vi "uc480_Sharpness_Measurement.vi"() -> ()   [LabVIEW 2011]
uses:
  C:/Program Files/Thorlabs/Scientific Imaging/DCx Camera Support/Develop/DotNet/uc480DotNet.dll
  Develop/DotNet/uc480DotNet.dll
panel:
  in  "Measuring Region":u32(ring) items=["Center", "Upper Left", "Upper Right", "Lower Left", "Lower Right"]
  in  "Zoom":enum32{"1:4", "1:2", "1:1", "2:1"}(radio)
  out "Sharpness":u32(slide) scale=0.0..100.0
  out "Image":picture
  in  "Camera ID":i32 min=0 max=255
  out "Serial Number":string
  out "AOI Height":i32=8
  out "AOI Width":i32=8
  out "Bits/Pixel":i32=8
  out "Error Out":errorcluster caption="error"
  in  "Exit Camera":bool
  in  "Init Camera":bool
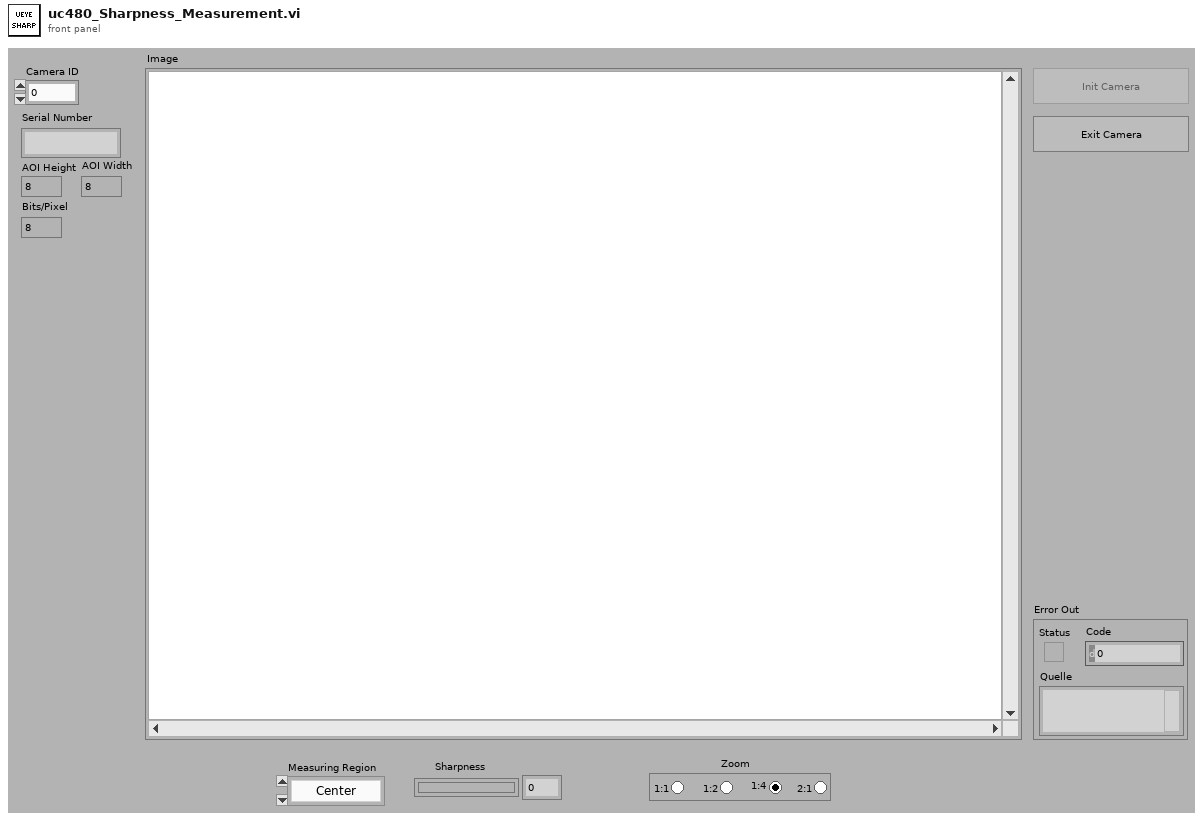
[diagram p1: front panel]
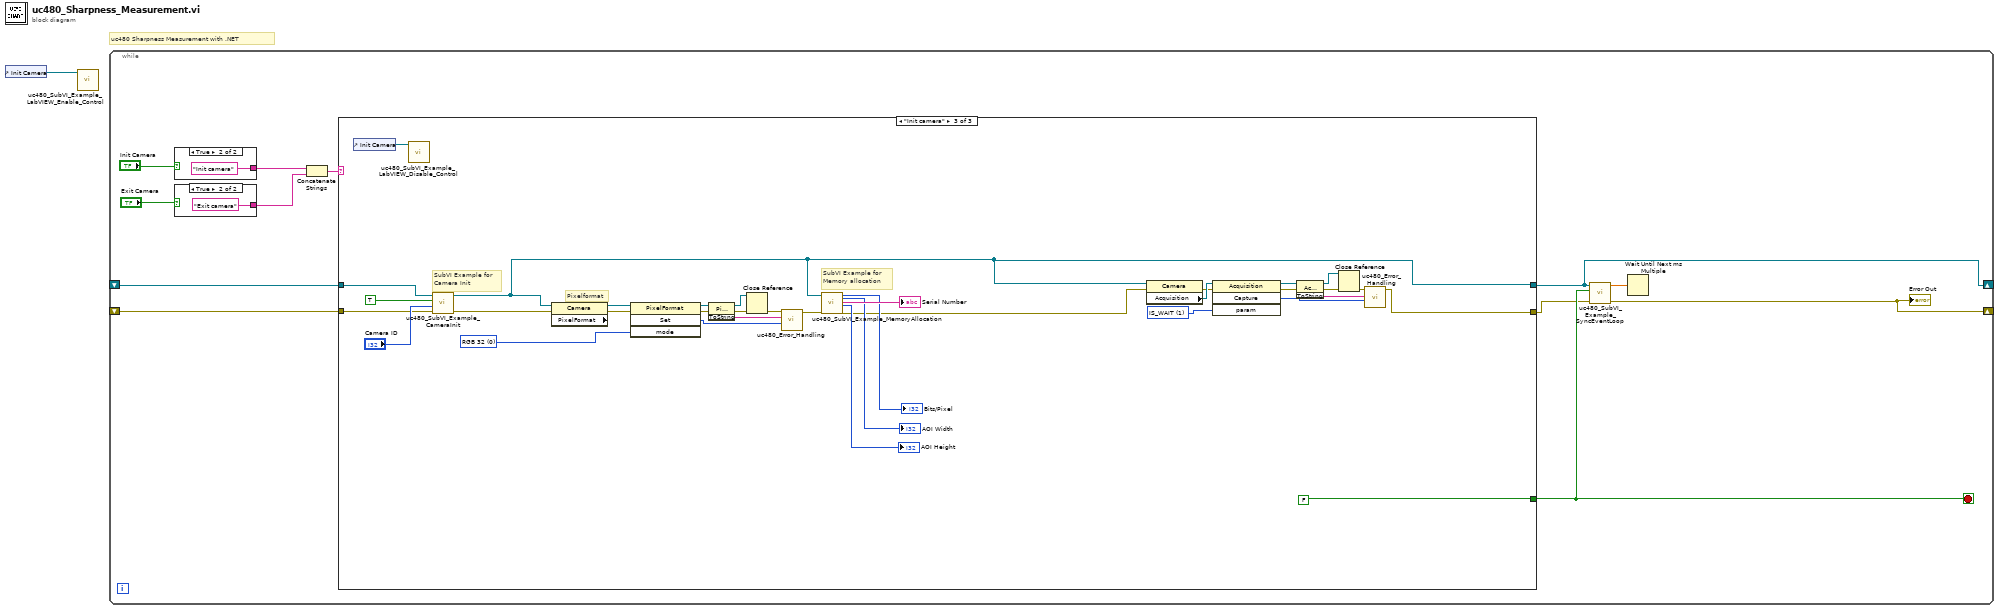
[diagram p0: block diagram]
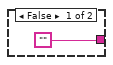
[diagram p2: hidden frame]
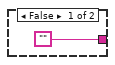
[diagram p3: hidden frame]
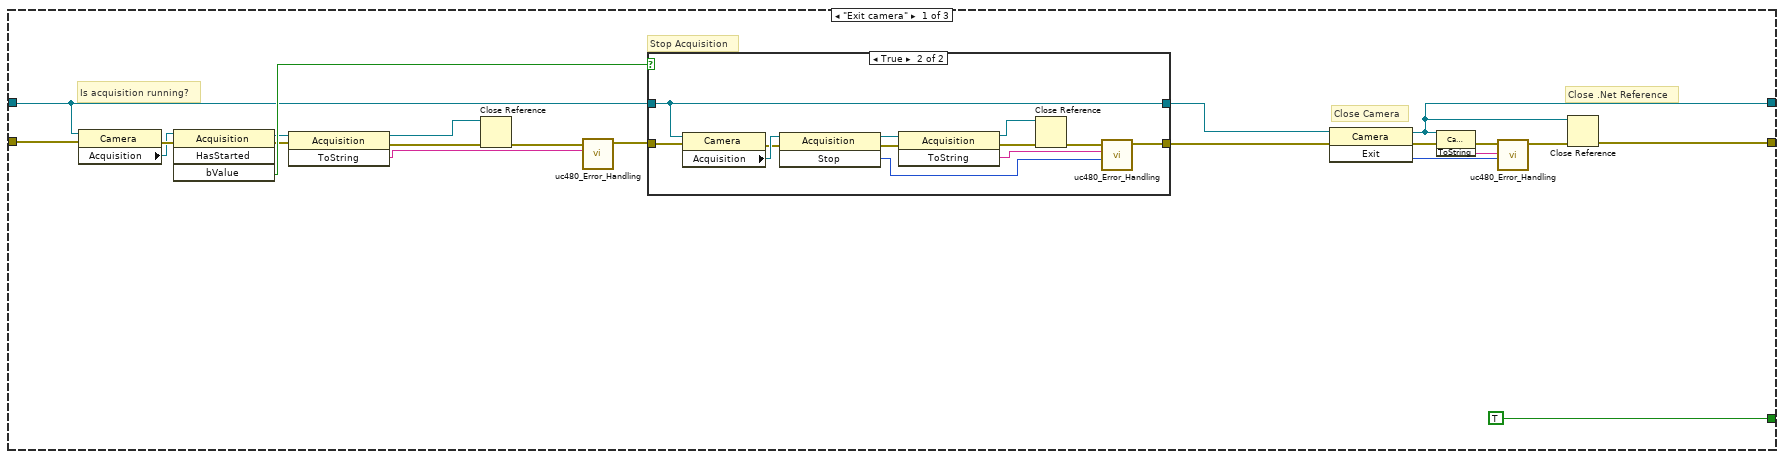
[diagram p4: hidden frame]
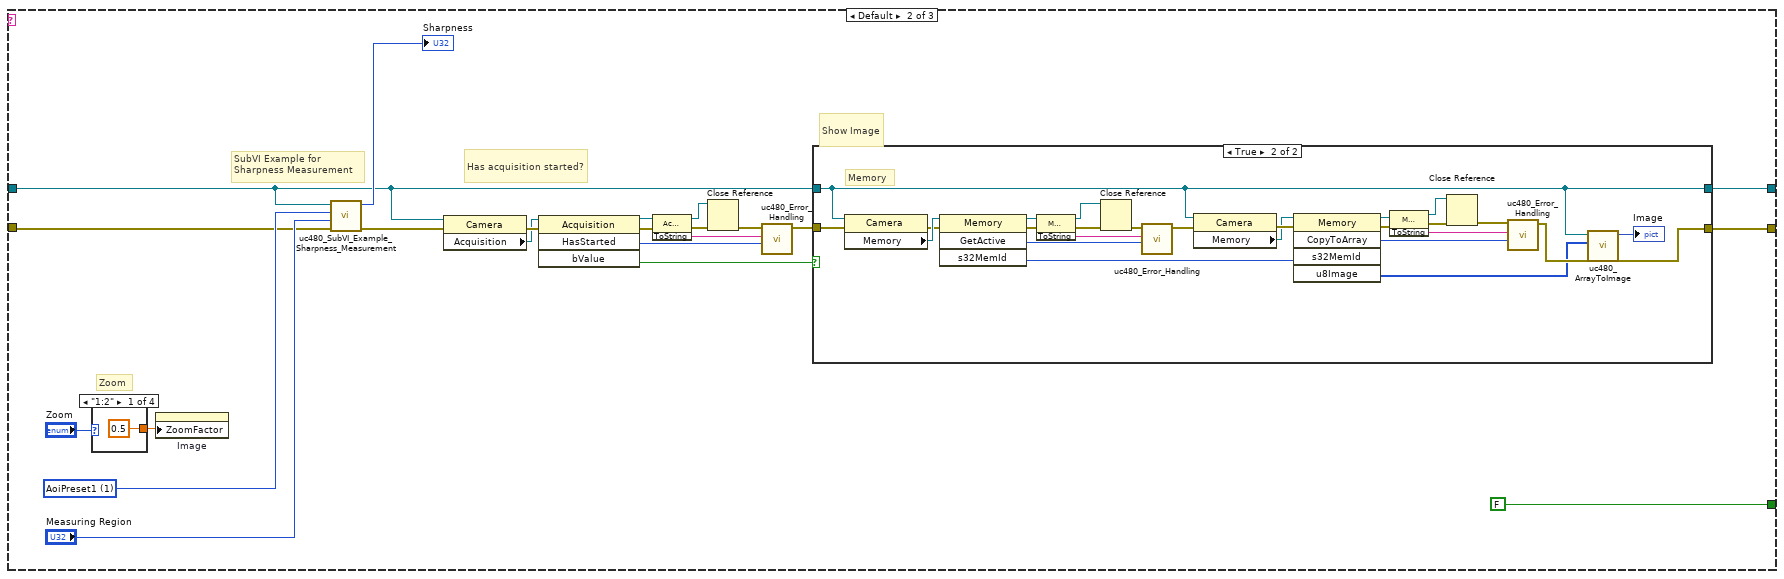
[diagram p6: hidden frame]
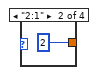
[diagram p7: hidden frame]
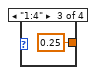
[diagram p8: hidden frame]
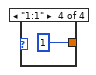
[diagram p9: hidden frame]
diagram:
  # "uc480 Sharpness Measurement with .NET"
  n1 = control-ref of="Init Camera"() -> (w1:refnum<vi>)
  n2 = call "uc480_SubVI_Example_LabVIEW_Enable_Control.vi"("UI Control (Reference)"=w1) -> ()  [unwired: 11 in]
  n3 = while {
    shift-right: [w3] -> _
    shift-left: _ -> [w8]
    shift-right: [w4] -> _
    shift-left: _ -> [w2]
    stop <- w7 stop-if-true
    n4 = case shown="True" "Init Camera" {
      tunnel: ["" "Init camera"] -> w12
      frame False {
      }
      frame True {
      }
    }
    n5 = case shown="True" "Exit Camera" {
      tunnel: ["" "Exit camera"] -> w9
      frame False {
      }
      frame True {
      }
    }
    n6 = Concatenate Strings(w12, w9) -> (w11:string)
    n7 = case shown="\"Init camera\"" w11 {
      tunnel: w2 -> [w23 w57 w134]
      tunnel: w8 -> [w24 w58 w133]
      tunnel: [w22 w66 w116] -> w4
      tunnel: [w21 w65 w117] -> w6
      tunnel: [TRUE FALSE FALSE] -> w7
      frame "Exit camera" {
        # "Close .Net Reference"
        # "Is acquisition running?"
        # "Stop Acquisition"
        # "Close Camera"
        n8 = property class="Camera"(reference=w23, error in=w24) -> (error out=w33:errorcluster, "Acquisition"=w32:refnum<k24>)  [unwired: 1 out]
        n9 = invoke class="Acquisition" method="HasStarted"(reference=w32, error in=w33) -> (reference out=w27:refnum<k24>, error out=w29:errorcluster, "bValue"=w31:bool)  [unwired: 2 in, 1 out]
        n10 = invoke class="Acquisition" method="ToString"(reference=w27, error in=w29) -> (reference out=w18:refnum<k24>, error out=w20:errorcluster, "ToString"=w28:string)  [unwired: 1 in]
        n11 = Close Reference(reference=w18, error in (no error)=w20) -> (error out=w19:errorcluster)
        n12 = call "uc480_Error_Handling.vi"("Error String"=w28, "Error In"=w19) -> ("Error Out"=w30:errorcluster)  [unwired: 9 in]
        n13 = case shown="True" w31 {
          tunnel: [w41 w52] -> w25
          tunnel: w30 -> [w41 w53]
          tunnel: w23 -> [w40 w45]
          tunnel: [w40 w45] -> w26
          frame False {
          }
          frame True {
            n14 = property class="Camera"(reference=w45, error in=w53) -> (error out=w49:errorcluster, "Acquisition"=w50:refnum<k24>)  [unwired: 1 out]
            n15 = invoke class="Acquisition" method="Stop"(reference=w50, error in=w49) -> (reference out=w47:refnum<k24>, error out=w48:errorcluster, "Stop"=w46:i32)  [unwired: 1 in]
            n16 = invoke class="Acquisition" method="ToString"(reference=w47, error in=w48) -> (reference out=w42:refnum<k24>, error out=w44:errorcluster, "ToString"=w51:string)  [unwired: 1 in]
            n17 = Close Reference(reference=w42, error in (no error)=w44) -> (error out=w43:errorcluster)
            n18 = call "uc480_Error_Handling.vi"("Error Code"=w46, "Error String"=w51, "Error In"=w43) -> ("Error Out"=w52:errorcluster)  [unwired: 8 in]
          }
        }
        n19 = invoke class="Camera" method="Exit"(reference=w26, error in=w25) -> (reference out=w22:refnum<k24>, error out=w36:errorcluster, "Exit"=w35:i32)  [unwired: 1 in]
        n20 = invoke class="Camera" method="ToString"(reference=w22, error in=w36) -> (error out=w37:errorcluster, "ToString"=w38:string)  [unwired: 1 in, 1 out]
        n21 = call "uc480_Error_Handling.vi"("Error Code"=w35, "Error String"=w38, "Error In"=w37) -> ("Error Out"=w34:errorcluster)  [unwired: 8 in]
        n22 = Close Reference ("Close Referenz")(reference=w22, error in (no error)=w34) -> (error out=w21:errorcluster)
      }
      frame Default {
        w61 = 1 items=["AoiPreset1"=1] ("ePreset")
        # "Zoom"
        # "SubVI Example for\nSharpness Measurement"
        # "Has acquisition started?"
        # "Show Image"
        n23 = case shown="\"1:2\"" "Zoom" {
          tunnel: [0.5 2 0.25 1] -> w63
          frame "1:2" {
          }
          frame "2:1" {
          }
          frame "1:4" {
          }
          frame "1:1" {
          }
        }
        n24 = property on="Image" class="Pict"("ZoomFactor"=w63) -> ()  [unwired: 2 in, 2 out]
        n25 = call "uc480_SubVI_Example_Sharpness_Measurement.vi"("Error In"=w58, "Measuring Region"="Measuring Region", "Preset"=w61, ".NET (Reference)"=w57) -> ("Error Out"=w59:errorcluster, "Sharpness"=→"Sharpness":u32)  [unwired: 6 in]
        n26 = property class="Camera"(reference=w57, error in=w59) -> (error out=w74:errorcluster, "Acquisition"=w73:refnum<k24>)  [unwired: 1 out]
        n27 = invoke class="Acquisition" method="HasStarted"(reference=w73, error in=w74) -> (reference out=w70:refnum<k24>, error out=w69:errorcluster, "HasStarted"=w68:i32, "bValue"=w72:bool)  [unwired: 2 in]
        n28 = invoke class="Acquisition" method="ToString"(reference=w70, error in=w69) -> (reference out=w54:refnum<k24>, error out=w56:errorcluster, "ToString"=w71:string)  [unwired: 1 in]
        n29 = Close Reference(reference=w54, error in (no error)=w56) -> (error out=w55:errorcluster)
        n30 = call "uc480_Error_Handling.vi"("Error Code"=w68, "Error String"=w71, "Error In"=w55) -> ("Error Out"=w67:errorcluster)  [unwired: 8 in]
        n31 = case shown="True" w72 {
          tunnel: [w81 w93] -> w65
          tunnel: w67 -> [w81 w92]
          tunnel: w57 -> [w80 w89]
          tunnel: [w80 w89] -> w66
          frame False {
          }
          frame True {
            # "Memory"
            n32 = property class="Camera"(reference=w89, error in=w92) -> (error out=w95:errorcluster, "Memory"=w96:refnum<k24>)  [unwired: 1 out]
            n33 = invoke class="Memory" method="GetActive"(reference=w96, error in=w95) -> (reference out=w101:refnum<k24>, error out=w100:errorcluster, "GetActive"=w102:i32, "s32MemId"=w94:i32)  [unwired: 2 in]
            n34 = invoke class="Memory" method="ToString"(reference=w101, error in=w100) -> (reference out=w85:refnum<k24>, error out=w87:errorcluster, "ToString"=w99:string)  [unwired: 1 in]
            n35 = Close Reference(reference=w85, error in (no error)=w87) -> (error out=w86:errorcluster)
            n36 = call "uc480_Error_Handling.vi"("Error Code"=w102, "Error String"=w99, "Error In"=w86) -> ("Error Out"=w103:errorcluster)  [unwired: 8 in]
            n37 = property class="Camera"(reference=w89, error in=w103) -> (error out=w98:errorcluster, "Memory"=w97:refnum<k24>)  [unwired: 1 out]
            n38 = invoke class="Memory" method="CopyToArray"(reference=w97, error in=w98, "s32MemId"=w94) -> (reference out=w105:refnum<k24>, error out=w106:errorcluster, "CopyToArray"=w107:i32, "u8Image"=w90:u8[])  [unwired: 2 in, 1 out]
            n39 = invoke class="Memory" method="ToString"(reference=w105, error in=w106) -> (reference out=w82:refnum<k24>, error out=w84:errorcluster, "ToString"=w104:string)  [unwired: 1 in]
            n40 = Close Reference(reference=w82, error in (no error)=w84) -> (error out=w83:errorcluster)
            n41 = call "uc480_Error_Handling.vi"("Error Code"=w107, "Error String"=w104, "Error In"=w83) -> ("Error Out"=w91:errorcluster)  [unwired: 8 in]
            n42 = call "uc480_ArrayToImage.vi"("Error In"=w91, "InArray"=w90, ".NET (Reference)"=w89) -> ("Error Out"=w93:errorcluster, "Image"=→"Image":picture)  [unwired: 7 in]
          }
        }
      }
      frame "Init camera" {
        w119 = 1 items=["IS_DONT_WAIT", "IS_WAIT"] ("Wait")
        w142 = 0 items=["RGB 32"=0, "RGB 24"=1, "Y8 Monochrom"=6] ("Mode")
        # "SubVI Example for \nMemory allocation"
        # "SubVI Example for \nCamera Init"
        # "Pixelformat"
        n43 = control-ref of="Init Camera"() -> (w115:refnum<vi>)
        n44 = call "uc480_SubVI_Example_LabVIEW_Disable_Control.vi"("UI Control (Reference)"=w115) -> ()  [unwired: 11 in]
        n45 = call "uc480_SubVI_Example_CameraInit.vi"("Error In"=w133, "Camera ID"="Camera ID", "Init Camera Flag"=TRUE, ".NET (Reference)"=w134) -> ("Error Out"=w139:errorcluster, ".NET (Reference)"=w116:refnum<k24>)  [unwired: 6 in]
        n46 = property class="Camera"(reference=w116, error in=w139) -> (error out=w140:errorcluster, "PixelFormat"=w141:refnum<k24>)  [unwired: 1 out]
        n47 = invoke class="PixelFormat" method="Set"(reference=w141, error in=w140, "mode"=w142) -> (reference out=w137:refnum<k24>, error out=w130:errorcluster, "Set"=w136:i32)  [unwired: 1 in, 1 out]
        n48 = invoke class="PixelFormat" method="ToString"(reference=w137, error in=w130) -> (reference out=w111:refnum<k24>, error out=w113:errorcluster, "ToString"=w138:string)  [unwired: 1 in]
        n49 = Close Reference(reference=w111, error in (no error)=w113) -> (error out=w112:errorcluster)
        n50 = call "uc480_Error_Handling.vi"("Error Code"=w136, "Error String"=w138, "Error In"=w112) -> ("Error Out"=w114:errorcluster)  [unwired: 8 in]
        n51 = call "uc480_SubVI_Example_MemoryAllocation.vi"(".NET (Reference)"=w116, "Error In"=w114) -> ("Bits/Pixel 2"=→"Bits/Pixel":i32, "Width"=→"AOI Width":i32, "Serial Number"=→"Serial Number":string, "Height"=→"AOI Height":i32, "Error Out"=w118:errorcluster)  [unwired: 13 in]
        n52 = property class="Camera"(reference=w116, error in=w118) -> (error out=w124:errorcluster, "Acquisition"=w125:refnum<k24>)  [unwired: 1 out]
        n53 = invoke class="Acquisition" method="Capture"(reference=w125, error in=w124, "param"=w119) -> (reference out=w121:refnum<k24>, error out=w122:errorcluster, "Capture"=w120:i32)  [unwired: 1 in, 1 out]
        n54 = invoke class="Acquisition" method="ToString"(reference=w121, error in=w122) -> (reference out=w108:refnum<k24>, error out=w110:errorcluster, "ToString"=w123:string)  [unwired: 1 in]
        n55 = Close Reference(reference=w108, error in (no error)=w110) -> (error out=w109:errorcluster)
        n56 = call "uc480_Error_Handling.vi"("Error Code"=w120, "Error String"=w123, "Error In"=w109) -> ("Error Out"=w117:errorcluster)  [unwired: 8 in]
      }
    }
    n57 = call "uc480_SubVI_Example_SyncEventLoop.vi"("Error In"=w6, "use sync"=w7, ".NET (Reference)"=w4) -> ("Error Out"=w3:errorcluster, "Synchronize (ms)"=w5:dbl)  [unwired: 7 in]
    "Error Out" <- w3
    n58 = Wait Until Next ms Multiple(millisecond multiple=w5) -> ()  [unwired: 1 out]
  }
